vi "get_all_raw_rates.vi"(8 "error in (no error)":errorcluster, 11 "VISA resource name":refnum<visa-resource-name>) -> (0 "error out":errorcluster, 2 "Rates (A/s)":dbl[](array[numeric]), 3 "VISA resource name out":refnum<visa-resource-name>)   [LabVIEW 2018]
doc: "Query all raw sensor rates in A/s. If sensor is not in use response will be 0."
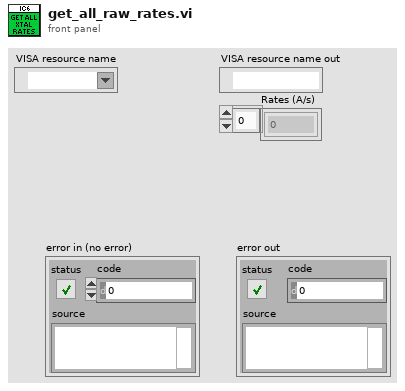
[diagram p1: front panel]
types:
  T1 = enum16{"Source", "General", "Input name", "Process name", "Logic", "Material", "Material name", "Output name", "Process", "Sensor", "Output type", "User message", "Layer", ""}
  T2 = enum16{"Hello", "Query", "Remote action", "Status", "Update"}
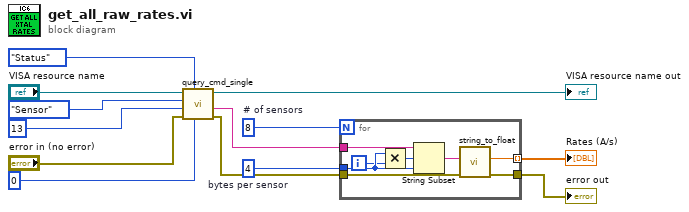
[diagram p0: block diagram]
diagram:
  w3 = 4  # bytes per sensor
  w4 = 8  # # of sensors
  n1 = call "query_cmd_single.vi"("Parameter"=u8 0 ("Sensor"), "Command group"=T2."Status", "error in (no error)"="error in (no error)", "Command ID"=u8 13, "Command subgroup"=T1."Sensor", "VISA resource name"="VISA resource name") -> ("error out"=w2:errorcluster, "formatted response"=w5:string, "VISA resource name out"=→"VISA resource name out":refnum<visa-resource-name>)  [unwired: 1 in, 2 out]
  n2 = for {
    N: w4 -> [_]
    tunnel: [w21] -> w1 mode=indexing
    tunnel: [w20] -> w7
    tunnel: w5 -> [w18]
    tunnel: w3 -> [w16]
    tunnel: w2 -> [w14]
    i -> [w15]
    n3 = Multiply(x=w16, y=w15) -> (x*y=w17:i32)
    n4 = String Subset(string=w18, offset (0)=w17, length (rest)=w16) -> (substring=w19:string)
    n5 = call "string_to_float.vi"("error in (no error)"=w14, "Float (string)"=w19) -> ("error out"=w20:errorcluster, "Float (sgl)"=w21:sgl)  [unwired: 8 in]
  }
  "error out" <- w7
  "Rates (A/s)" <- w1
